vi "Test Encode and Decode.vi"() -> ()   [LabVIEW 2020]
uses:
  Image Type.ctl
  Image Comparison/Image Comparison.lvclass
panel:
  out "length 2":i32
  out "length":i32
  out "Image 2 (Encoded Image)":picture
  out "Image 1 (Original Image)":picture
  out "Composite Score":dbl
  out "Bytes of Encoded Data":i32
  out "Encoded Data Correct?":bool
  in  "Image File Type":T1
  # "More the better"
  # "Closer to Zero (0) the better"
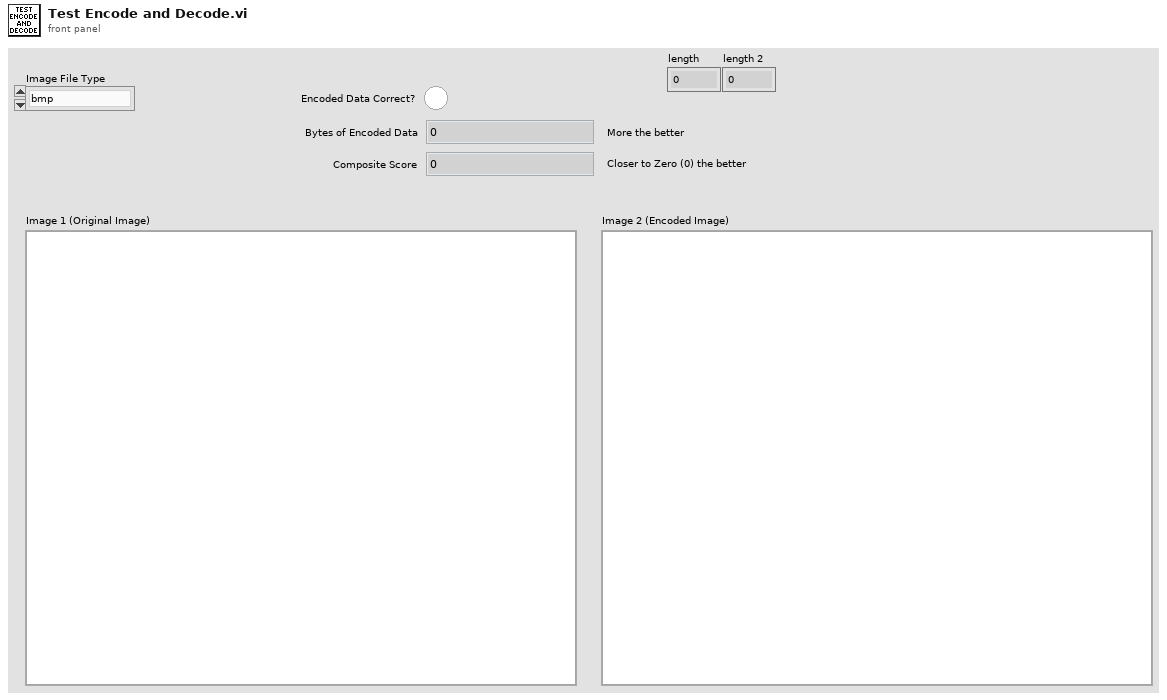
[diagram p1: front panel]
types:
  T1 = typedef "Image Type.ctl" = enum16{"bmp", "jpg", "png"}
  T2 = typedef "imagedata.ctl" = cluster{"image type":i32, "image depth":i32, "image":u8[], "mask":u8[], "colors":u32[], "Rectangle":cluster{"left":i16, "top":i16, "right":i16, "bottom":i16}}
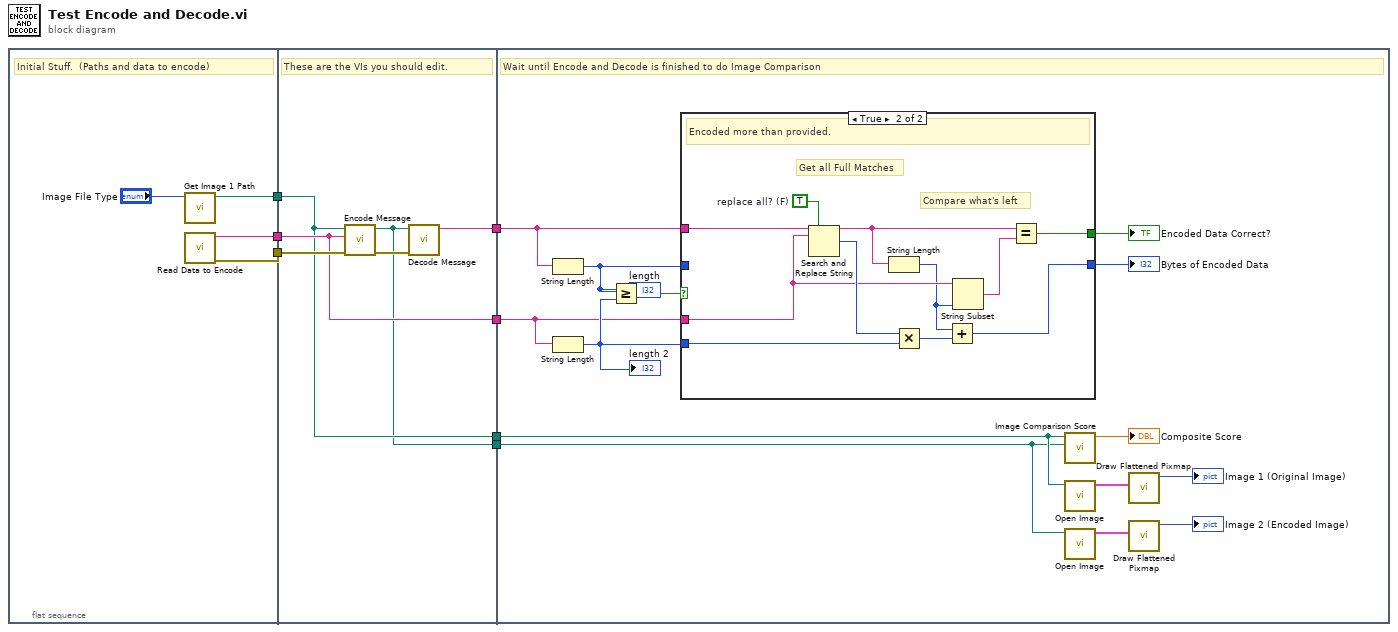
[diagram p0: block diagram]
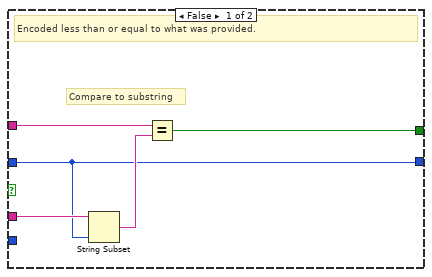
[diagram p2: hidden frame]
diagram:
  n1 = flat-sequence {
    tunnel: [w8] -> w3
    tunnel: [w10] -> w2
    tunnel: [w9] -> w1
    tunnel: [w12] -> w7
    tunnel: [w15] -> w6
    tunnel: [w14] -> w5
    tunnel: [w13] -> w4
    tunnel: w3 -> [w15]
    tunnel: w2 -> [w14]
    tunnel: w1 -> [w16]
    tunnel: w7 -> [w29]
    tunnel: w6 -> [w18]
    tunnel: w5 -> [w25]
    tunnel: w4 -> [w24]
    frame #0 {
      # "Initial Stuff.  (Paths and data to encode)"
      n2 = call "Get Image 1 Path.vi"("Image File Type"="Image File Type") -> ("Image 1 Path out"=w10:path)  [unwired: 10 in]
      n3 = call "Read Data to Encode.vi"() -> ("error out"=w9:errorcluster, "Data to Encode"=w8:string)  [unwired: 10 in]
    }
    frame #1 {
      # "These are the VIs you should edit."
      n4 = call "Encode Message.vi"("Error In"=w16, "Message In"=w15, "Image 1 Path in"=w14) -> ("Error Out"=w17:errorcluster, "Image 2 Path out"=w13:path)  [unwired: 7 in]
      n5 = call "Decode Message.vi"("Error In"=w17, "Image 2 Path in"=w13) -> ("Decoded Message"=w12:string)  [unwired: 8 in, 1 out]
    }
    frame #2 {
      # "Wait until Encode and Decode is finished to do Image Comparison"
      n6 = String Length(string=w29) -> (length=w30:i32)
      "length" <- w30
      n7 = String Length(string=w18) -> (length=w19:i32)
      "length 2" <- w19
      n8 = Greater Or Equal?(x=w30, y=w19) -> (x >= y?=w31:bool)
      n9 = case shown="True" w31 {
        tunnel: w18 -> [w36 w43]
        tunnel: w30 -> [w32 _]
        tunnel: w29 -> [w35 w47]
        tunnel: [w33 w40] -> w28
        tunnel: [w32 w37] -> w27
        tunnel: w19 -> [_ w44]
        frame False {
          # "Compare to substring"
          # "Encoded less than or equal to what was provided."
          n10 = String Subset(string=w36, length (rest)=w32) -> (substring=w34:string)  [unwired: 1 in]
          n11 = Equal?(x=w35, y=w34) -> (x = y?=w33:bool)
        }
        frame True {
          w46 = TRUE  # replace all? (F)
          # "Compare what's left"
          # "Get all Full Matches"
          # "Encoded more than provided."
          n12 = Search and Replace String(replace all?=w46, input string=w47, search string=w43) -> (result string=w42:string, number of replacements=w45:i32)  [unwired: 5 in, 2 out]
          n13 = String Length(string=w42) -> (length=w39:i32)
          n14 = Multiply(x=w45, y=w44) -> (x*y=w38:i32)
          n15 = Add(x=w39, y=w38) -> (x+y=w37:i32)
          n16 = String Subset(string=w43, length (rest)=w39) -> (substring=w41:string)  [unwired: 1 in]
          n17 = Equal?(x=w42, y=w41) -> (x = y?=w40:bool)
        }
      }
      "Encoded Data Correct?" <- w28
      "Bytes of Encoded Data" <- w27
      n18 = call "Image Comparison Score.vi"("Image 2"=w24, "Image 1"=w25) -> ("Composite Score"=→"Composite Score":dbl)  [unwired: 9 in]
      n19 = call "Open Image.vi"("Image"=w25) -> ("image data"=w23:T2)  [unwired: 9 in, 1 out]
      n20 = call "Open Image.vi"("Image"=w24) -> ("image data"=w21:T2)  [unwired: 9 in, 1 out]
      n21 = call <vilib>:"Draw Flattened Pixmap.vi"("image data"=w23) -> ("new picture"=→"Image 1 (Original Image)":picture)  [unwired: 8 in]
      n22 = call <vilib>:"Draw Flattened Pixmap.vi"("image data"=w21) -> ("new picture"=→"Image 2 (Encoded Image)":picture)  [unwired: 8 in]
    }
  }
